vi "Init Check.vi"(11 "Actor in":refnum<class "Actor.lvclass">) -> (2 "Not initialized?":bool)   [LabVIEW 2020, in "Actor Framework.lvlib" / "Actor.lvclass"]
uses:
  Actor.lvclass
  Message Priority Queue/Message Priority Queue.lvclass
  Message Enqueuer/Message Enqueuer.lvclass
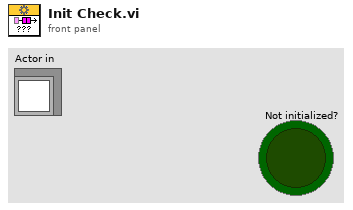
[diagram p1: front panel]
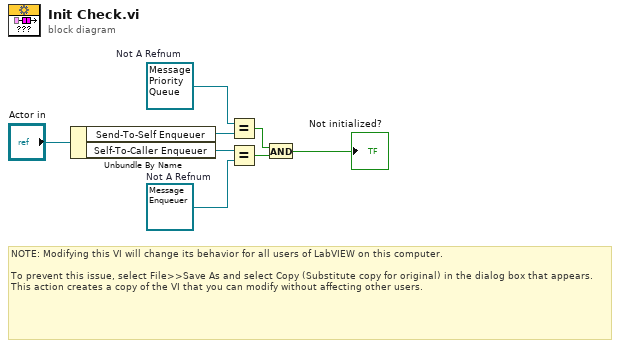
[diagram p0: block diagram]
diagram:
  w4 = refnum<class "Message Enqueuer.lvclass"> refnum  # Not A Refnum
  w7 = refnum<class "Message Priority Queue.lvclass"> refnum  # Not A Refnum
  # "NOTE: Modifying this VI will change its behavior for all users of LabVIEW on this computer.\n\nTo prevent this issue, select File>>Save As and select Copy (Substitute copy for original) in the dialog box that appears. This action creates a copy of the VI that you can modify without affecting other users."
  n1 = Unbundle By Name("Actor in") -> ("Send-To-Self Enqueuer"=w6:refnum<class "Message Priority Queue.lvclass">, "Self-To-Caller Enqueuer"=w5:refnum<class "Message Enqueuer.lvclass">)
  n2 = Equal?(x=w7, y=w6) -> (x = y?=w3:bool)
  n3 = Equal?(x=w5, y=w4) -> (x = y?=w2:bool)
  n4 = And(x=w3, y=w2) -> (x .and. y?=→"Not initialized?":bool)
